vi "OnDataChange.vi"(0 "DataProcessor in":refnum<class "DataProcessor.lvclass">, 1 "DataExchange":T1, 3 "error in (no error)":errorcluster) -> (7 "DataProcessor out":refnum<class "DataProcessor.lvclass">, 10 "error out":errorcluster)   [LabVIEW 2020, in "DataProcessor.lvlib" / "DataProcessor.lvclass"]
uses:
  DataProcessor.lvclass
  Hardware Abstraction Layer/Component/Device/Device/DataExchange.ctl
  <vilib>/ActorFramework/Message Enqueuer/Message Enqueuer.lvclass
  DataProcessor.lvclass/DataProcessor.ctl
  Interface/DataListener Messages/OnDataChange Msg/OnDataChange Msg.lvclass/OnDataChange Msg.ctl
  <vilib>/ActorFramework/Message Enqueuer/Message Enqueuer.lvclass/Message Enqueuer.ctl
  <vilib>/ActorFramework/Message Enqueuer/Enqueue.vi
  Interface/DataListener Messages/OnDataChange Msg/OnDataChange Msg.lvclass
  C:/Program Files/National Instruments/LabVIEW 2020/vi.lib/ActorFramework/Message/Message.lvclass
  <vilib>/ActorFramework/Message Priority Queue/Priority Enqueue.vi
  Interface/DataListener/DataListener.lvclass
panel:
  in  "Enqueuer":refnum<class "Message Enqueuer.lvclass">
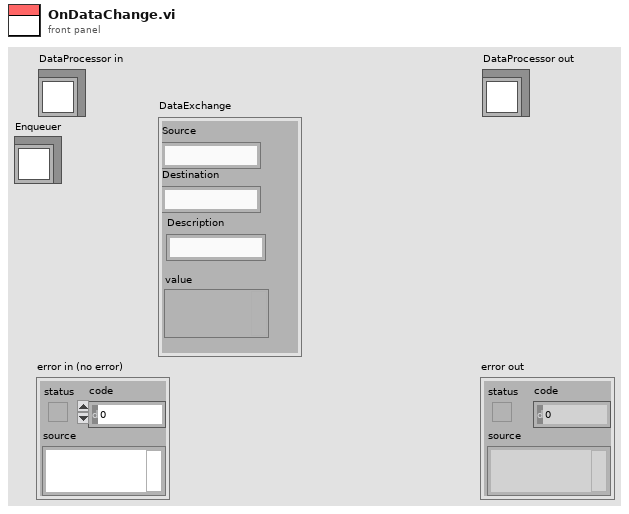
[diagram p1: front panel]
types:
  T1 = typedef "DataListener.lvclass/DataExchange.ctl" = cluster{"Source":string, "Destination":string, "Description":string, "value":variant}
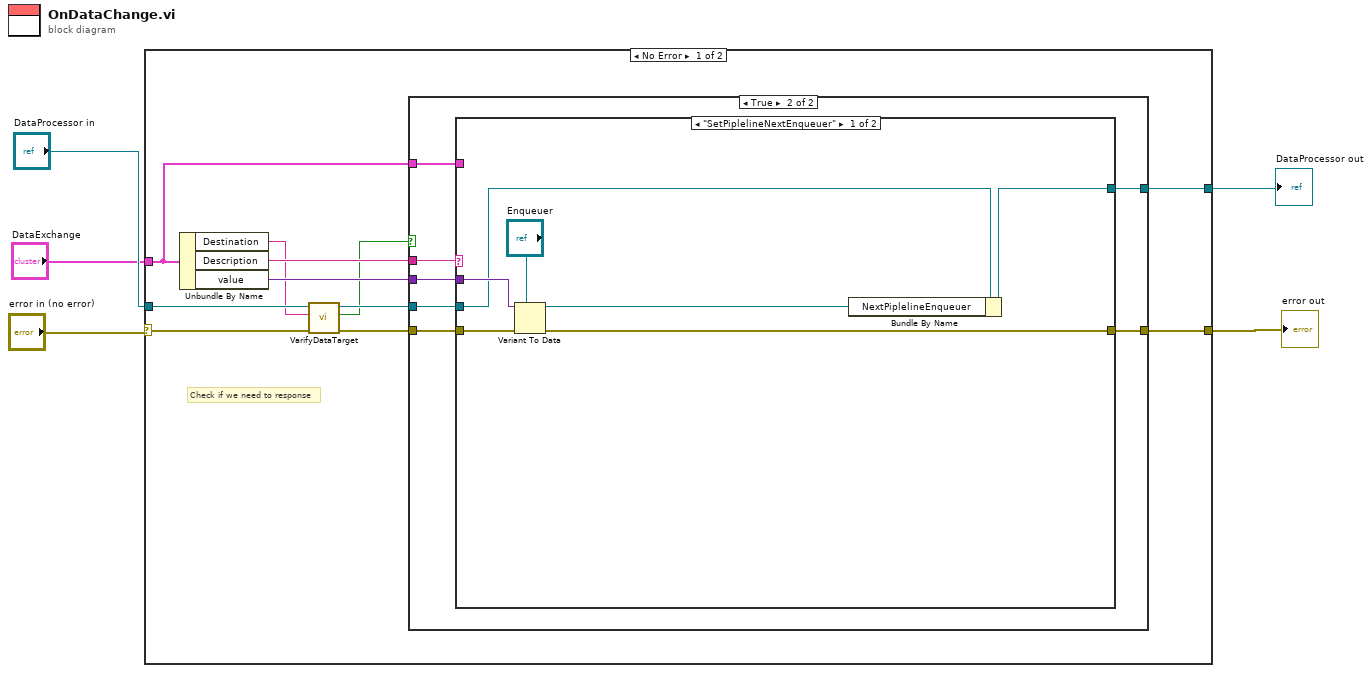
[diagram p0: block diagram]
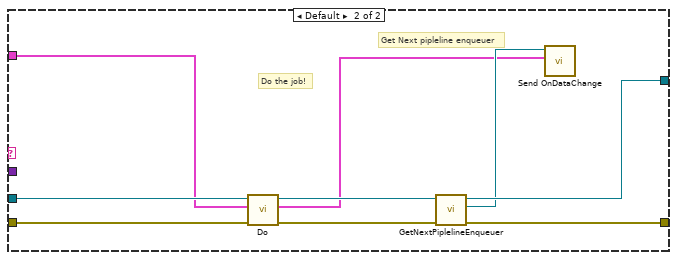
[diagram p3: hidden frame]
diagram:
  n1 = case shown="No Error" "error in (no error)" {
    selector: "error in (no error)" -> [w14 w43]
    tunnel: [w15 w43] -> w2
    tunnel: "DataProcessor in" -> [w10 w42]
    tunnel: [w16 w42] -> w1
    tunnel: "DataExchange" -> [w8 _]
    frame No Error {
      # "Check if we need to response"
      n2 = Unbundle By Name(w8) -> ("Destination"=w7:string, "Description"=w13:string, "value"=w12:variant)
      n3 = call-dynamic "VarifyDataTarget.vi"("error in (no error)"=w14, "Destination"=w7, "DataProcessor in"=w10) -> ("error out"=w11:errorcluster, "Response?"=w6:bool, "DataProcessor out"=w9:refnum<class "DataProcessor.lvclass">)  [unwired: 6 in]
      n4 = case shown="True" w6 {
        tunnel: [w18 w25] -> w16
        tunnel: w9 -> [w18 w22]
        tunnel: [w17 w23] -> w15
        tunnel: w11 -> [w17 w24]
        tunnel: w13 -> [_ w20]
        tunnel: w12 -> [_ w19]
        tunnel: w8 -> [_ w21]
        frame False {
        }
        frame True {
          n5 = case shown="\"SetPiplelineNextEnqueuer\"" w20 {
            tunnel: [w27 w41] -> w25
            tunnel: w24 -> [w32 w40]
            tunnel: [w31 w39] -> w23
            tunnel: w22 -> [w28 w35]
            tunnel: w21 -> [_ w34]
            tunnel: w19 -> [w30 _]
            frame "SetPiplelineNextEnqueuer" {
              n6 = Variant To Data(error in=w32, type="Enqueuer", Variant=w30) -> (data=w26:refnum<class "Message Enqueuer.lvclass">, error out=w31:errorcluster)
              n7 = Bundle By Name(cluster=w28, "NextPiplelineEnqueuer"=w26) -> (w27:refnum<class "DataProcessor.lvclass">)
            }
            frame Default {
              # "Do the job!"
              # "Get Next pipleline enqueuer"
              n8 = call-dynamic "Do.vi"("error in (no error)"=w40, "DataExchange"=w34, "DataProcessor in"=w35) -> ("error out"=w37:errorcluster, "DataExchange Out"=w33:T1, "DataProcessor out"=w36:refnum<class "DataProcessor.lvclass">)  [unwired: 6 in]
              n9 = call-dynamic "GetNextPiplelineEnqueuer.vi"("error in (no error)"=w37, "DataProcessor in"=w36) -> ("error out"=w39:errorcluster, "NextPiplelineEnqueuer"=w38:refnum<class "Message Enqueuer.lvclass">, "DataProcessor out"=w41:refnum<class "DataProcessor.lvclass">)  [unwired: 7 in]
              n10 = call "Send OnDataChange.vi"("DataExchange"=w33, "Message Enqueuer"=w38) -> ()  [unwired: 8 in, 2 out]
            }
          }
        }
      }
    }
    frame Error {
    }
  }
  "error out" <- w2
  "DataProcessor out" <- w1
